vi "Sleep Until Future Time.vi"(7 "FTE Limits (ns)":T1={"Maximum"=200000000, "Minimum"=10000} {"Maximum" format="%.0e"; "Minimum" format="%.0e"}, 8 "error in (no error)":errorcluster, 10 "Wake Offset":i64=2000, 11 "Wake Time (ns)":i64) -> (0 "error out":errorcluster, 2 "Wake Time (ns)":i64, 3 "Sleep TIme":i64)   [LabVIEW 2021, in "Time_CIF_U.lvlib"]
doc: "This will put the task to sleep until the configured wake time is reached. \n\nWake Time is the system time in TIA (ns).\n\nWake Offset will subract from the wake time to wake earlier. This allows tuning the wake on the system to account for execution time. \n\nFTE (Future Time Event) limits provides a maximum and minimum limit for sleep for the loop. If the calculated sleep duration is beyond the maximum future time event this will wake early and give a warning. If the wake time is before the minimum it will skip sleep. \n\nWake Time is the actual time when the loop woke. \n\nSleep Time is the actual time when the loop slept. If sleep was skipped these are set corrrectly to allow determining idle/sleep time."
uses:
  Time_CIF_U.lvlib
  Typedef/Future Time Event Limits.ctl
  Typedef/Errors.ctl
  LabVIEW Time to TAI Time.vi
  Errors/Append Error Location.vi
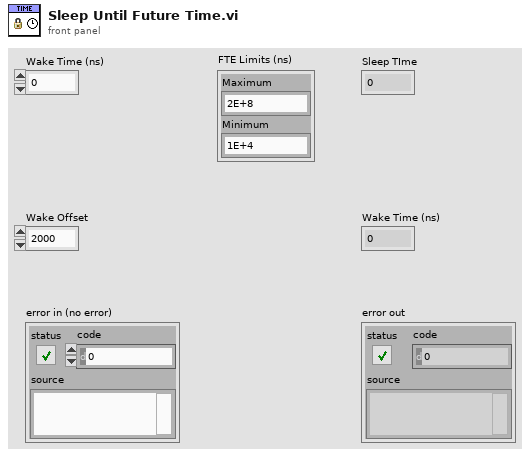
[diagram p1: front panel]
types:
  T1 = typedef "Time_CIF_U.lvlib/Future Time Event Limits.ctl" = cluster{"Maximum":i64, "Minimum":i64}
  T2 = typedef "Time_CIF_U.lvlib/Errors.ctl" = enum16{"Clock ID Match", "Invalid Clock ID", "Long Sleep"}
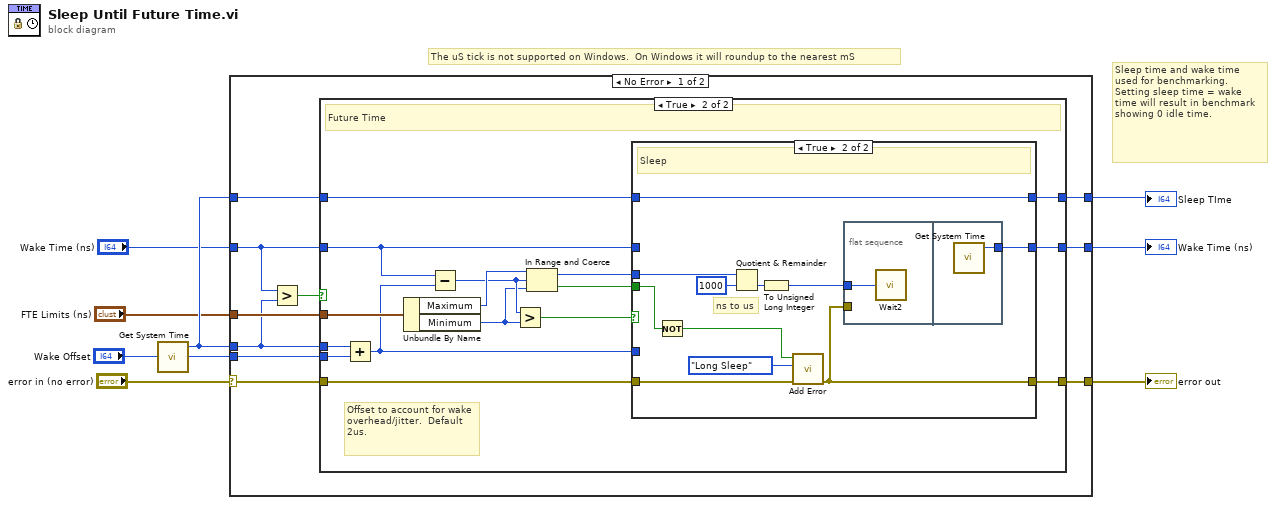
[diagram p0: block diagram]
diagram:
  # "Sleep time and wake time used for benchmarking.  Setting sleep time = wake time will result in benchmark showing 0 idle time."
  # "The uS tick is not supported on Windows.  On Windows it will roundup to the nearest mS"
  n1 = call "Get System Time.vi"() -> ("Time (ns)"=w8:i64)  [unwired: 5 in]
  n2 = case shown="No Error" "error in (no error)" {
    selector: "error in (no error)" -> [w15 w55]
    tunnel: "Wake Time (ns)" -> [w18 w54]
    tunnel: w8 -> [w9 _]
    tunnel: [w14 w55] -> w3
    tunnel: "FTE Limits (ns)" -> [w16 _]
    tunnel: "Wake Offset" -> [w10 _]
    tunnel: [w13 w54] -> w2
    tunnel: [w11 w53] -> w1
    tunnel: w8 -> [w12 w53]
    frame No Error {
      n3 = Greater?(x=w18, y=w9) -> (0:w17:bool)
      n4 = case shown="True" w17 {
        tunnel: w18 -> [_ w26]
        tunnel: w16 -> [_ w36]
        tunnel: w15 -> [w20 w33]
        tunnel: [w20 w32] -> w14
        tunnel: [w19 w27] -> w13
        tunnel: w12 -> [w19 w25]
        tunnel: [w19 w24] -> w11
        tunnel: w10 -> [_ w23]
        tunnel: w9 -> [_ w22]
        frame False {
          # "Past time, no sleep"
        }
        frame True {
          # "Offset to account for wake overhead/jitter.  Default 2us."
          # "Future Time"
          n5 = Add(x=w22, y=w23) -> (x+y=w21:i64)
          n6 = Unbundle By Name(w36) -> ("Maximum"=w35:i64, "Minimum"=w30:i64)
          n7 = Subtract(x=w26, y=w21) -> (x-y=w31:i64)
          n8 = Greater?(x=w31, y=w30) -> (0:w29:bool)
          n9 = In Range and Coerce(upper limit=w35, x=w31, lower limit=w30) -> (coerced(x)=w34:i64, In Range?=w28:bool)
          n10 = case shown="True" w29 {
            tunnel: w34 -> [_ w49]
            tunnel: w33 -> [w39 w46]
            tunnel: [w39 w47] -> w32
            tunnel: w28 -> [_ w48]
            tunnel: [w38 w43] -> w27
            tunnel: w26 -> [w38 _]
            tunnel: w25 -> [w37 w42]
            tunnel: [w37 w42] -> w24
            tunnel: w21 -> [_ _]
            frame False {
              # "Used to provide correct idle time stats"
              # "Sleep less than minimum"
            }
            frame True {
              # "ns to us"
              # "Sleep"
              n11 = Not(x=w48) -> (.not. x?=w45:bool)
              n12 = Quotient & Remainder(x=w49, y=i64 1000) -> (floor(x/y)=w40:i64)  [unwired: 1 out]
              n13 = To Unsigned Long Integer(number=w40) -> (unsigned 32bit integer=w41:u32)
              n14 = call "Add Error.vi"("error in (no error)"=w46, "Error"=Errors."Long Sleep", "Insert Error"=w45) -> ("error out"=w47:errorcluster)  [unwired: 8 in]
              n15 = flat-sequence {
                tunnel: w41 -> [w51]
                tunnel: w47 -> [_]
                tunnel: [w52] -> w43
                frame #0 {
                  n16 = call "Wait2"("Count(uSec)"=w51) -> ()  [unwired: 1 out]
                }
                frame #1 {
                  n17 = call "Get System Time.vi"() -> ("Time (ns)"=w52:i64)  [unwired: 5 in]
                }
              }
            }
          }
        }
      }
    }
    frame Error {
    }
  }
  "error out" <- w3
  "Wake Time (ns)" <- w2
  "Sleep TIme" <- w1
